vi "DestroyBase.vi"(0 "reference in":refnum<class "G#RealTimeTemplate.lvclass">, 5 "error in (no error)":errorcluster) -> (14 "reference out":refnum<class "G#RealTimeTemplate.lvclass">, 19 "error out":errorcluster)   [LabVIEW 2020, in "G#RealTimeTemplate.lvclass"]
doc: "Destructor."
uses:
  G#RealTimeTemplate.lvclass
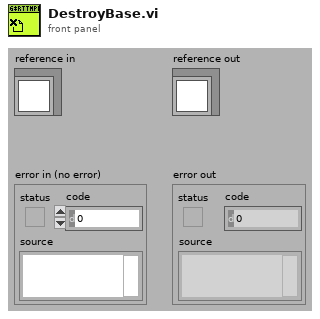
[diagram p1: front panel]
types:
  T1 = typedef "G#RealTimeTemplate.lvclass/ObjectAttributes.ctl" = cluster{"MyAttribute":dbl}
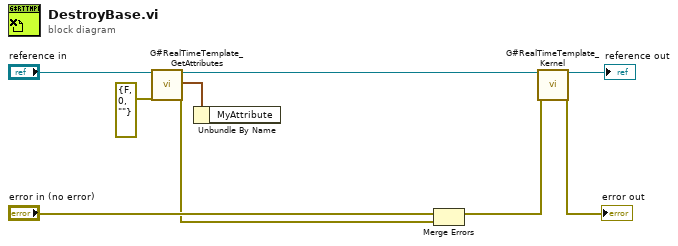
[diagram p0: block diagram]
diagram:
  n1 = call "G#RealTimeTemplate_GetAttributes.vi"("reference in"="reference in", "error in (no error)"=errorcluster {"status"=FALSE, "code"=0, "source"=""}) -> ("reference out"=w4:refnum<class "G#RealTimeTemplate.lvclass">, "attributes"=w5:T1, "error out"=w8:errorcluster)  [unwired: 14 in, 1 out]
  n2 = Unbundle By Name(w5) -> ()  [unwired: 1 out]
  n3 = Merge Errors("error in (no error)", w8) -> (w2:errorcluster)
  n4 = call "G#RealTimeTemplate_Kernel.vi"("reference in"=w4, "error in (no error)"=w2) -> ("reference out"=→"reference out":refnum<class "G#RealTimeTemplate.lvclass">, "error out"=→"error out":errorcluster)  [unwired: 16 in]
